vi "Polar Plot - Data.vi"(5 "Scale Polar plot":dbl=0.2, 6 "Size":u16=1, 7 "Lines/Points":enum16{"Lines", "Points"}(ring)=enum."Points", 8 "polar attributes":T1, 9 "grid measurements":T2, 10 "data array [mag, phase (deg)]":cluster{"magnitude":dbl, "phase":dbl}[](array[cluster]), 11 "new picture in":picture) -> (2 "Position":cluster{i16, i16}[](array[cluster]), 3 "new picture out":picture)   [LabVIEW 2020]
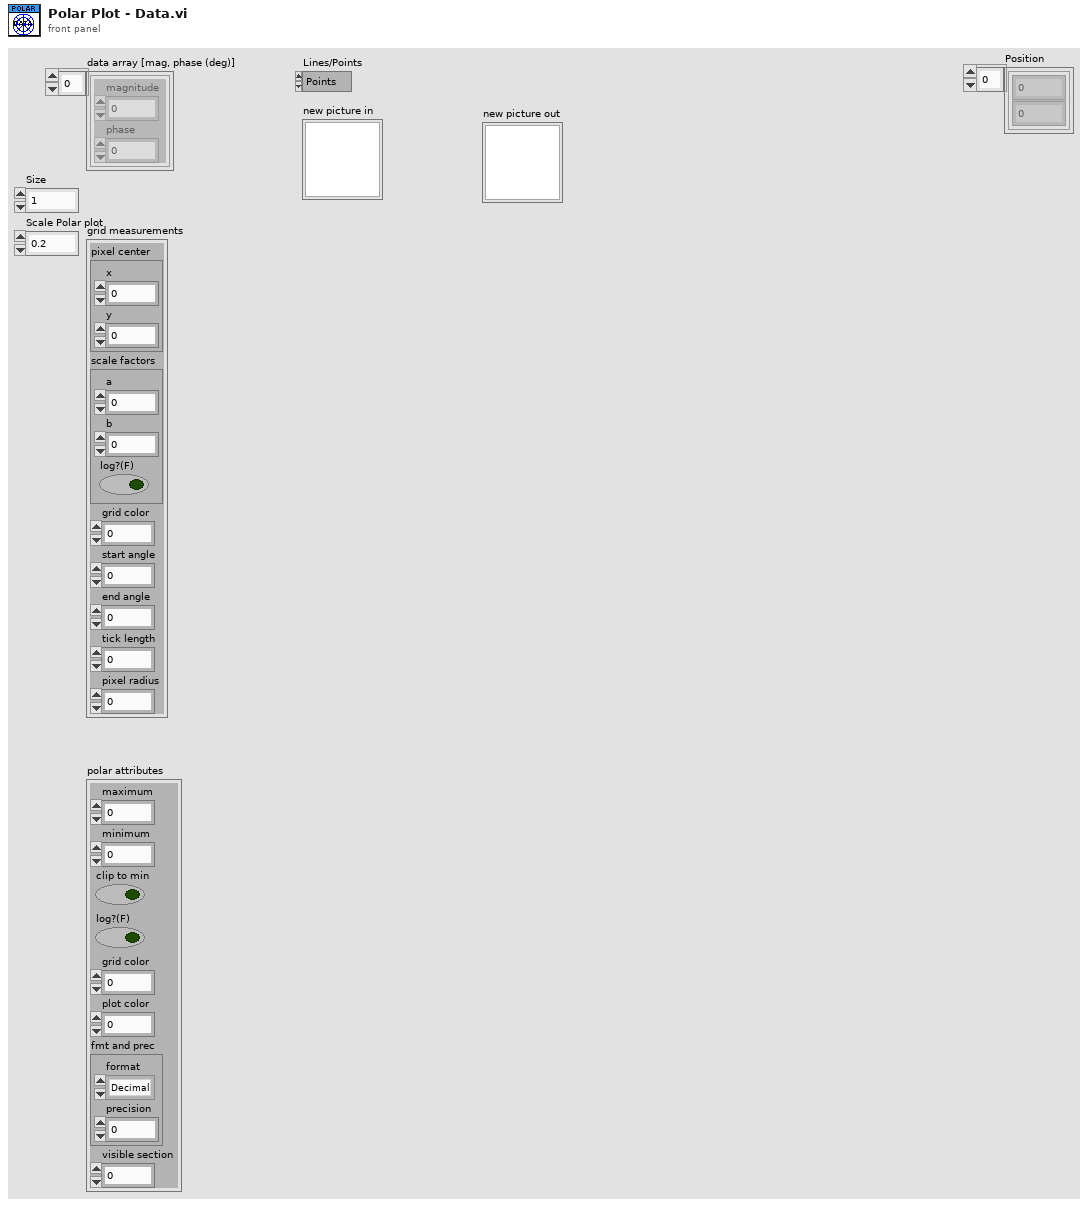
[diagram p1: front panel]
types:
  T1 = cluster{"maximum":dbl, "minimum":dbl, "clip to min":bool, "log?(F)":bool, "grid color":u32, "plot color":u32, "fmt and prec":cluster{"format":enum8{"Decimal", "Scientific", "Engineering", "Binary", "Octal", "Hex"}, "precision":u8}, "visible section":u16}
  T2 = cluster{"pixel center":cluster{"x":i16, "y":i16}, "scale factors":cluster{"a":dbl, "b":dbl, "log?(F)":bool}, "grid color":u32, "start angle":dbl, "end angle":dbl, "tick length":i16, "pixel radius":i32}
  T3 = enum32{"Solid", "Dash", "Dot", "DashDot", "DashDotDot"}
  T4 = cluster{"Size":u16, "Style":enum32{"Solid", "Dash", "Dot", "DashDot", "DashDotDot"}}
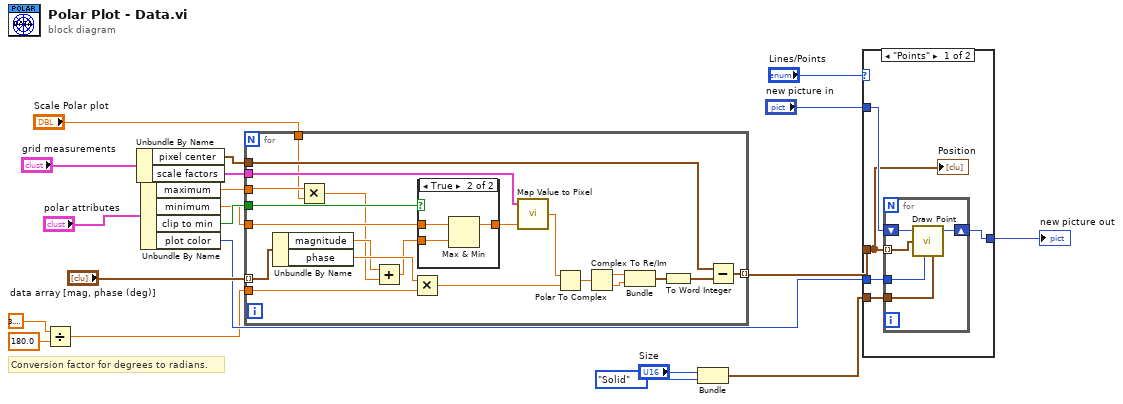
[diagram p0: block diagram]
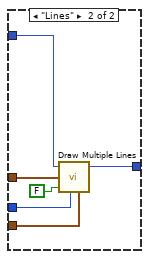
[diagram p2: hidden frame]
diagram:
  # "Conversion factor for degrees to radians."
  n1 = Divide(x=3.141592653589793, y=180.0) -> (x/y=w10:dbl)
  n2 = Unbundle By Name("grid measurements") -> ("pixel center"=w6:cluster{"x":i16, "y":i16}, "scale factors"=w5:cluster{"a":dbl, "b":dbl, "log?(F)":bool})
  n3 = Unbundle By Name("polar attributes") -> ("maximum"=w2:dbl, "minimum"=w7:dbl, "clip to min"=w8:bool, "plot color"=w13:u32)
  n4 = for {
    tunnel: "data array [mag, phase (deg)]" -> [w41] mode=indexing
    tunnel: w6 -> [w40]
    tunnel: [w39] -> w12 mode=indexing
    tunnel: w5 -> [w34]
    tunnel: w7 -> [w31]
    tunnel: w8 -> [w30]
    tunnel: w10 -> [w27]
    tunnel: w2 -> [w24]
    tunnel: "Scale Polar plot" -> [w21]
    n5 = Unbundle By Name(w41) -> ("magnitude"=w25:dbl, "phase"=w28:dbl)
    n6 = Multiply(x=w24, y=w21) -> (x*y=w23:dbl)
    n7 = Add(x=w25, y=w23) -> (x+y=w22:dbl)
    n8 = Multiply(x=w28, y=w27) -> (x*y=w29:dbl)
    n9 = case shown="True" w30 {
      tunnel: w22 -> [w42 w45]
      tunnel: [w42 w44] -> w32
      tunnel: w31 -> [_ w43]
      frame False {
      }
      frame True {
        n10 = Max & Min(x=w43, y=w45) -> (max(x,y)=w44:dbl)  [unwired: 1 out]
      }
    }
    n11 = call <vilib>:"Map Value to Pixel.vi"("x"=w32, "scale factors"=w34) -> ("pixel"=w33:dbl)  [unwired: 1 out]
    n12 = Polar To Complex(1:w29, 2:w33) -> (0:w38:cdb)
    n13 = Complex To Re/Im(x + iy=w38) -> (x=w36:dbl, y=w26:dbl)
    n14 = Bundle(w36, w26) -> (w37:cluster{dbl, dbl})  [unwired: 1 out]
    n15 = To Word Integer(number=w37) -> (16bit integer=w35:cluster{i16, i16})
    n16 = Subtract(x=w40, y=w35) -> (x-y=w39:cluster{i16, i16})
  }
  n17 = Bundle("Size"="Size", "Style"=T3."Solid") -> (w16:T4)  [unwired: 1 in]
  n18 = case shown="\"Points\"" "Lines/Points" {
    tunnel: w12 -> [w46 w60]
    tunnel: w13 -> [w48 w59]
    tunnel: [w49 w58] -> w19
    tunnel: "new picture in" -> [w50 w57]
    tunnel: w16 -> [w47 w56]
    frame "Points" {
      n19 = for {
        tunnel: w46 -> [w55] mode=indexing
        shift-right: [w53] -> w49
        shift-left: w50 -> [w54]
        tunnel: w48 -> [w52]
        tunnel: w47 -> [w51]
        n20 = call <vilib>:"Draw Point.vi"("picture"=w54, "point(x,y)"=w55, "color(black)"=w52, "pen"=w51) -> ("new picture"=w53:picture)  [unwired: 5 out]
      }
      "Position" <- w46
    }
    frame "Lines" {
      n21 = call <vilib>:"Draw Multiple Lines.vi"("picture"=w57, "line endpoints"=w60, "fill?(F)"=FALSE, "color(black)"=w59, "pen"=w56) -> ("new picture"=w58:picture)  [unwired: 4 out]
    }
  }
  "new picture out" <- w19
